vi "Write Background noise.vi"(8 "error in (no error)":errorcluster, 10 "Background noise":u32[](array[numeric]), 11 "Processing in":refnum<class "Processing.lvclass">) -> (0 "error out":errorcluster, 3 "Processing out":refnum<class "Processing.lvclass">)   [LabVIEW 2014, in "Processing.lvclass"]
uses:
  Processing.lvclass
  Processing.lvclass/Processing.ctl
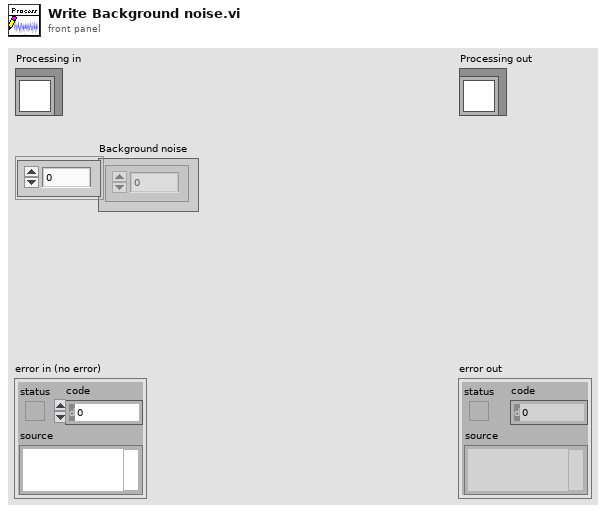
[diagram p1: front panel]
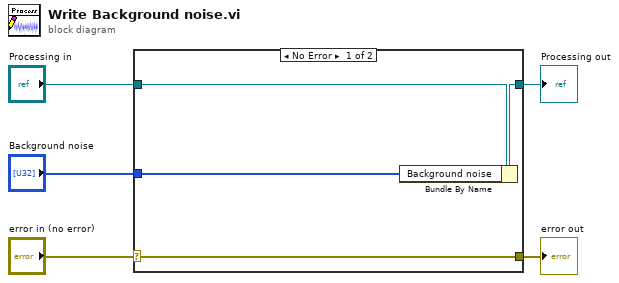
[diagram p0: block diagram]
diagram:
  n1 = case shown="No Error" "error in (no error)" {
    selector: "error in (no error)" -> [w9 w10]
    tunnel: [w9 w10] -> w4
    tunnel: [w7 w11] -> w2
    tunnel: "Processing in" -> [w8 w11]
    tunnel: "Background noise" -> [w6 _]
    frame No Error {
      n2 = Bundle By Name(cluster=w8, "Background noise"=w6) -> (w7:refnum<class "Processing.lvclass">)
    }
    frame Error {
    }
  }
  "error out" <- w4
  "Processing out" <- w2
